vi "swabian_convert_rawdata_to_photons.vi"(0 "Raw_data_file":path, 5 "output_data_file":path, 7 "sync_channel":i32, 9 "sync_period_ps":u64, 11 "error in (no error)":errorcluster) -> (15 "error out":errorcluster)   [LabVIEW 2018]
uses:
  cmake-build-release/swabian_lib.dll
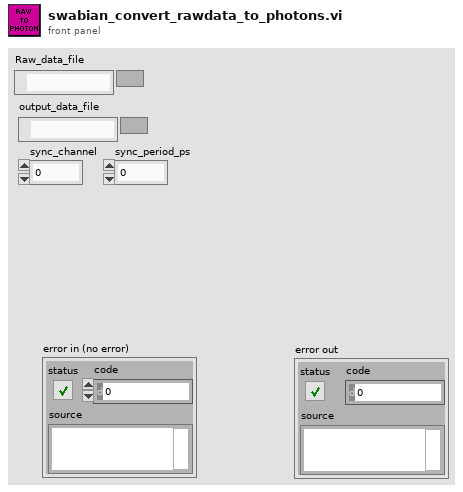
[diagram p1: front panel]
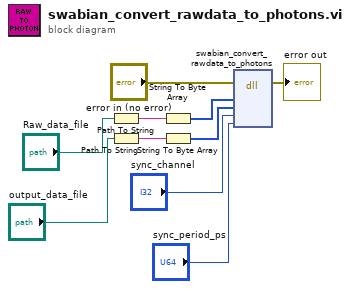
[diagram p0: block diagram]
diagram:
  n1 = Path To String(path="Raw_data_file") -> (string=w7:string)
  n2 = Path To String(path="output_data_file") -> (string=w5:string)
  n3 = String To Byte Array(string=w7) -> (unsigned byte array=w6:u8[])
  n4 = String To Byte Array(string=w5) -> (unsigned byte array=w3:u8[])
  n5 = dll-call lib="C:/Users/bspoka/Documents/swabian_LV/swabian_vis/swabian_lib/cmake-build-release/swabian_lib.dll" fn="swabian_convert_rawdata_to_photons"(error in="error in (no error)", "raw_filepath"=w6, "output_filepath"=w3, "sync_channel"="sync_channel", "sync_rate"="sync_period_ps") -> (error out=→"error out":errorcluster)  [unwired: 7 in, 1 out]
